vi "GPSMODBUSTCP解析.vi"(11 "Registers":u16[](array[numeric])) -> (3 "GPS解析":T1={"定位状态"=TRUE, "卫星数量"=0, "时间标识"=timestamp(0 s since 1904-01-01), "纬度"=0.0, "南北"="", "经度"=0.0, "东西"=""} {"经度" format="%#.6g"; "纬度" format="%#.6g"})   [LabVIEW 2016, in "环境动力监测库.lvlib" / "NMEA.lvlib"]
uses:
  NMEA.lvlib
  <vilib>/Utility/miscctls.llb/LVDateTimeRec.ctl
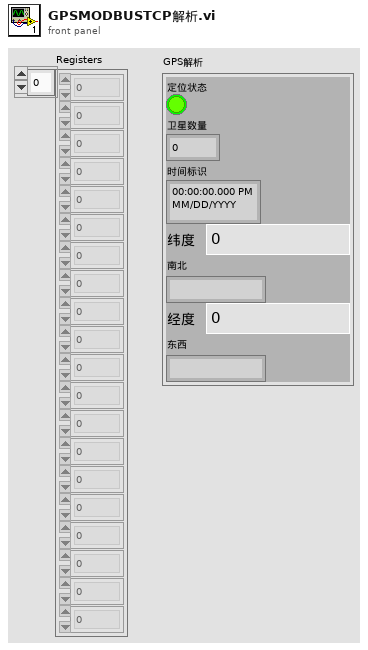
[diagram p1: front panel]
types:
  T1 = cluster{"定位状态":bool, "卫星数量":u16, "时间标识":timestamp, "纬度":dbl, "南北":string, "经度":dbl, "东西":string}
  T2 = typedef "LVDateTimeRec.ctl" = cluster{"fractional second":dbl, "second":i32, "minute":i32, "hour":i32, "day of month":i32, "month":i32, "year":i32, "day of week":i32, "day of year":i32, "DST":i32}
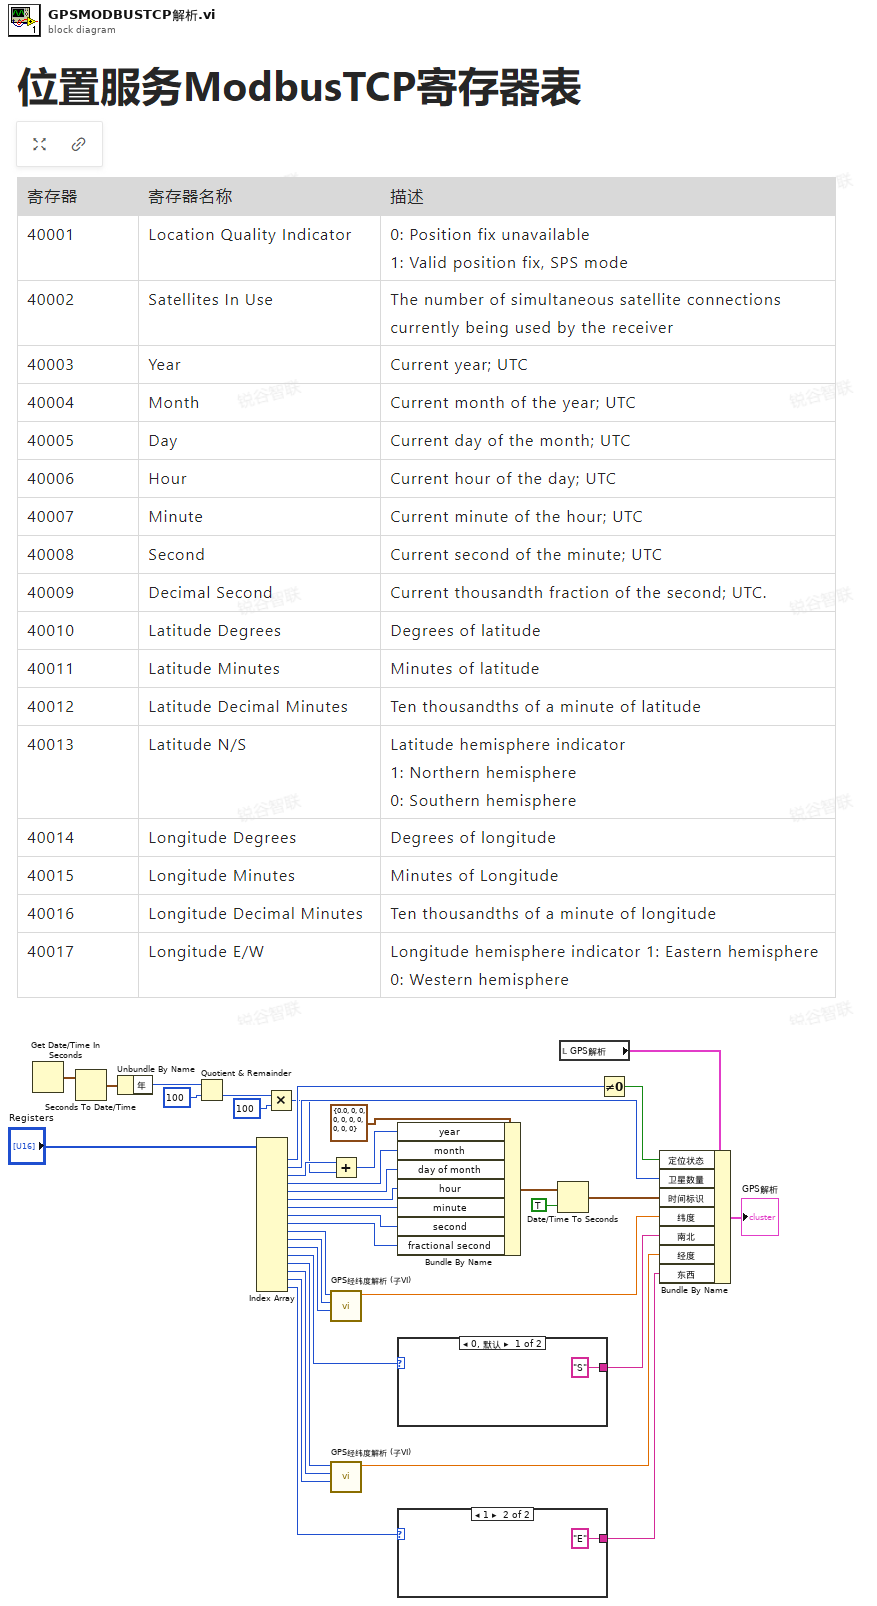
[diagram p0: block diagram]
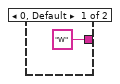
[diagram p2: hidden frame]
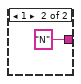
[diagram p3: hidden frame]
diagram:
  n1 = Get Date/Time In Seconds() -> (seconds since 1Jan1904=w19:timestamp)
  n2 = Seconds To Date/Time(time stamp (now)=w19) -> (date time rec=w18:T2)  [unwired: 1 in]
  n3 = Unbundle By Name(w18) -> ("年"=w17:i32)
  n4 = Quotient & Remainder(x=w17, y=100) -> (floor(x/y)=w15:i32)  [unwired: 1 out]
  n5 = Index Array(array="Registers") -> (element #1=w36:u16, element #2=w32:u16, element #3=w21:u16, element #4=w30:u16, element #5=w28:u16, element #6=w27:u16, element #7=w26:u16, element #8=w25:u16, element #9=w24:u16, element #10=w2:u16, element #11=w3:u16, element #12=w4:u16, element #13=w11:u16, element #14=w10:u16, element #15=w7:u16, element #16=w6:u16, element #17=w9:u16)  [unwired: 17 in]
  n6 = Multiply(x=w15, y=100) -> (x*y=w13:i32)
  n7 = Add(x=w21, y=w13) -> (x+y=w20:i32)
  n8 = call "GPS经纬度解析 (子VI).vi"("小数"=w4, "分"=w3, "度"=w2) -> ("数值输出"=w1:dbl)  [unwired: 8 in]
  n9 = call "GPS经纬度解析 (子VI).vi"("小数"=w6, "分"=w7, "度"=w10) -> ("数值输出"=w5:dbl)  [unwired: 8 in]
  n10 = Bundle By Name(cluster=T2 {"fractional second"=0.0, "second"=0, "minute"=0, "hour"=0, "day of month"=0, "month"=0, "year"=0, "day of week"=0, "day of year"=0, "DST"=0} ("日期时间记录"), "year"=w20, "month"=w30, "day of month"=w28, "hour"=w27, "minute"=w26, "second"=w25, "fractional second"=w24) -> (w23:T2)
  n11 = case shown="0, 默认" w11 {
    tunnel: ["S" "N"] -> w12
    frame 0, Default {
    }
    frame 1 {
    }
  }
  n12 = case shown="1" w9 {
    tunnel: ["W" "E"] -> w8
    frame 0, Default {
    }
    frame 1 {
    }
  }
  n13 = Date/Time To Seconds(1:TRUE ("是UTC (F)"), 2:w23) -> (0:w22:timestamp)
  n14 = local read "GPS解析"() -> (w35:T1)
  n15 = Not Equal To 0?(x=w36) -> (x != 0?=w34:bool)
  n16 = Bundle By Name(cluster=w35, "定位状态"=w34, "卫星数量"=w32, "时间标识"=w22, "纬度"=w1, "南北"=w12, "经度"=w5, "东西"=w8) -> (→"GPS解析":T1)
